vi "ex_9.vi"() -> ()   [LabVIEW 2020]
panel:
  out "String OUT":string
  in  "String IN":string
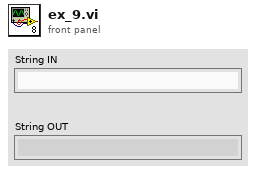
[diagram p1: front panel]
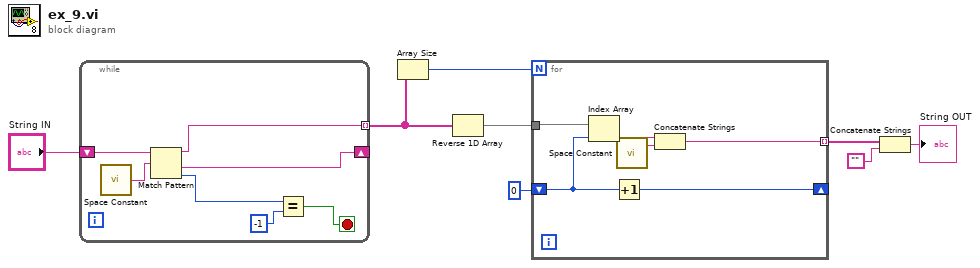
[diagram p0: block diagram]
diagram:
  n1 = while {
    tunnel: [w9] -> w8 mode=indexing
    shift-right: [w10] -> _
    shift-left: "String IN" -> [w15]
    stop <- w11 stop-if-true
    n2 = call <vilib>:"Space Constant.vi"() -> ("String"=w14:string)
    n3 = Match Pattern(string=w15, regular expression=w14) -> (before substring=w9:string, after substring=w10:string, offset past match=w13:i32)  [unwired: 1 in, 1 out]
    n4 = Equal?(x=w13, y=-1) -> (x = y?=w11:bool)
  }
  n5 = Array Size(array=w8) -> (size(s)=w4:i32)
  n6 = Reverse 1D Array(array=w8) -> (reversed array=w6:string[])
  n7 = for {
    N: w4 -> [_]
    tunnel: w6 -> [w19]
    shift-right: [w21] -> _
    shift-left: 0 -> [w20]
    tunnel: [w16] -> w3 mode=indexing
    n8 = Index Array(array=w19, index=w20) -> (element=w18:string)
    n9 = Increment(x=w20) -> (x+1=w21:i32)
    n10 = call <vilib>:"Space Constant.vi"() -> ("String"=w17:string)
    n11 = Concatenate Strings(w18, w17) -> (w16:string)
  }
  n12 = Concatenate Strings(w3, "") -> (→"String OUT":string)
